vi "Auto 5.vi"(8 "Error In":errorcluster) -> (0 "Error Out":errorcluster)   [LabVIEW 2014]
uses:
  Robot Global Data.vi
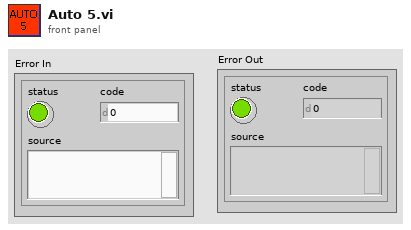
[diagram p1: front panel]
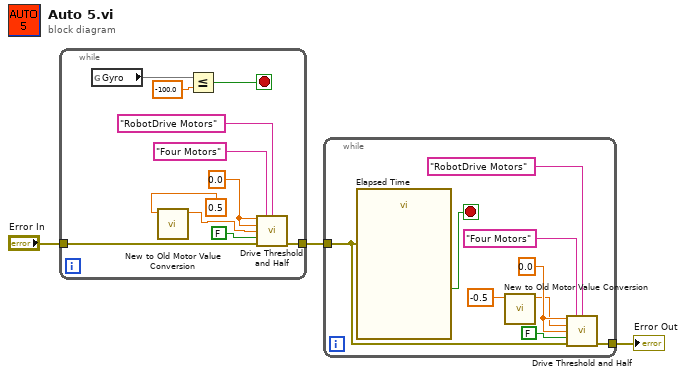
[diagram p0: block diagram]
diagram:
  n1 = while {
    tunnel: "Error In" -> [w11]
    tunnel: [w10] -> w3
    stop <- w6 stop-if-true
    w9 = 0.0 ("Arm Value")
    n2 = global read "Robot Global Data.vi" "Gyro"() -> (w8)
    n3 = call "New to Old Motor Value Conversion.vi"("Motor Value In"=0.5 ("X In")) -> ("New to Old Conversion Value Out"=w4:dbl)  [unwired: 9 in, 1 out]
    n4 = Less Or Equal?(x=w8, y=-100.0) -> (x <= y?=w6:bool)
    n5 = call "Drive Threshold and Half.vi"("X In"=w9, "Drive refnum name"="Four Motors" ("refnum name"), "Send to DB Name"="RobotDrive Motors" ("Name"), "Y In"=w9, "R In"=w4, "Speed Toggle"=FALSE ("Grabber Open/Close"), "Error In"=w11) -> ("Error Out"=w10:errorcluster)  [unwired: 8 in]
  }
  n6 = while {
    tunnel: w3 -> [w17]
    tunnel: [w20] -> w2
    stop <- w18 stop-if-true
    w19 = 0.0 ("Arm Value")
    n7 = call "Elapsed Time"("error in (no error)"=w17) -> ("Time has Elapsed"=w18:bool)  [unwired: 11 in, 7 out]
    n8 = call "New to Old Motor Value Conversion.vi"("Motor Value In"=-0.5 ("X In")) -> ("New to Old Conversion Value Out"=w15:dbl)  [unwired: 9 in, 1 out]
    n9 = call "Drive Threshold and Half.vi"("X In"=w19, "Drive refnum name"="Four Motors" ("refnum name"), "Send to DB Name"="RobotDrive Motors" ("Name"), "Y In"=w15, "R In"=w19, "Speed Toggle"=FALSE ("Grabber Open/Close"), "Error In"=w17) -> ("Error Out"=w20:errorcluster)  [unwired: 8 in]
  }
  "Error Out" <- w2
